vi "Rotation Application Settings.vi"() -> ()   [LabVIEW 2012]
panel:
  in  "Simulated Stage Settings":T1
  in  "Rotation Initialization Settings":T2={"Final Angle (degrees)"=45.0, "Polynomial Degree (n)"=1.0, "Number of Rotation Steps"=4500}
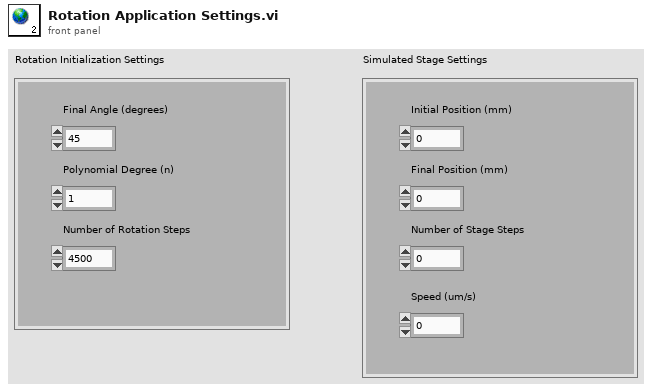
[diagram p1: front panel]
types:
  T1 = cluster{"Initial Position (mm)":dbl, "Final Position (mm)":dbl, "Number of Stage Steps":dbl, "Speed (um/s)":dbl}
  T2 = cluster{"Final Angle (degrees)":dbl, "Polynomial Degree (n)":dbl, "Number of Rotation Steps":u32}
diagram:
